vi "Get or Add Sheet.vi"(8 "error in":errorcluster, 10 "Sheet Name":string, 11 "SpreadsheetDoc in":refnum<k24>) -> (0 "error out":errorcluster, 1 "Sheet Index":i32, 2 "Sheet":refnum<k24>, 3 "SpreadsheetDoc out":refnum<k24>)   [LabVIEW 2021, in "Open Xml.lvlib"]
uses:
  Open Xml.lvlib
  D:/git/Open-Xml-LabVIEW/dll/DocumentFormat.OpenXml.dll
  dll/DocumentFormat.OpenXml.dll
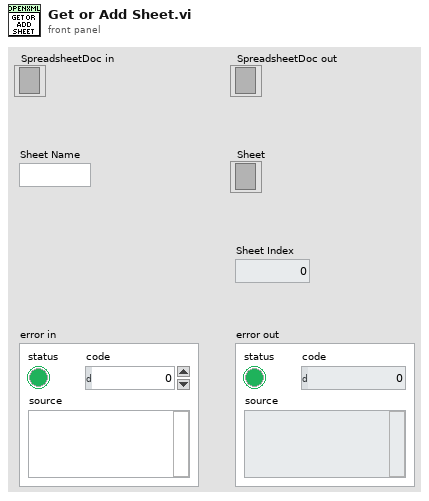
[diagram p1: front panel]
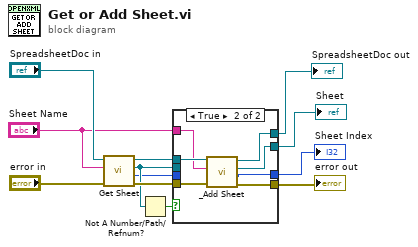
[diagram p0: block diagram]
diagram:
  n1 = call "Get Sheet.vi"("error in"="error in", "SheetName"="Sheet Name", "SpreadsheetDoc in"="SpreadsheetDoc in") -> ("error out"=w11:errorcluster, "Sheet Index"=w1:i32, "Sheet"=w7:refnum<k24>, "SpreadsheetDoc out"=w6:refnum<k24>)  [unwired: 5 in]
  n2 = Not A Number/Path/Refnum?(number/path/refnum=w7) -> (NaN/Path/Refnum?=w8:bool)
  n3 = case shown="True" w8 {
    tunnel: [w14 w23] -> w12
    tunnel: w11 -> [w14 w22]
    tunnel: w7 -> [w16 _]
    tunnel: w6 -> [w15 w21]
    tunnel: [w15 w20] -> w5
    tunnel: "Sheet Name" -> [_ w19]
    tunnel: [w16 w18] -> w3
    tunnel: [w13 w17] -> w2
    tunnel: w1 -> [w13 _]
    frame False {
    }
    frame True {
      n4 = call "_Add Sheet.vi"("error in"=w22, "SheetName"=w19, "SpreadsheetDoc in"=w21) -> ("error out"=w23:errorcluster, "Sheet Index"=w17:i32, "Sheet"=w18:refnum<k24>, "SpreadsheetDoc out"=w20:refnum<k24>)  [unwired: 5 in]
    }
  }
  "error out" <- w12
  "Sheet" <- w3
  "SpreadsheetDoc out" <- w5
  "Sheet Index" <- w2
